vi "SCPI_Log.vi"(11 "SCOP Log In":T1(ring)) -> (3 "SCPI Log Out":string)   [LabVIEW 2009]
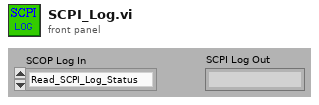
[diagram p1: front panel]
types:
  T1 = enum16{"Read_SCPI_Log_Status", "No_SCPI_Log", "Log_SCPI", "Reset"}
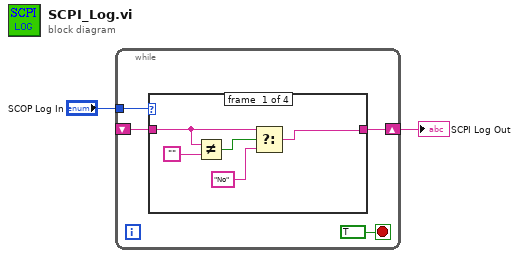
[diagram p0: block diagram]
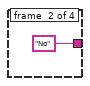
[diagram p2: hidden frame]
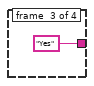
[diagram p3: hidden frame]
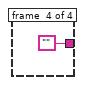
[diagram p4: hidden frame]
diagram:
  n1 = while {
    shift-right: [w5] -> w1
    shift-left: _ -> [w4]
    tunnel: "SCOP Log In" -> [w6]
    stop <- TRUE stop-if-true
    n2 = case shown="\"Read_SCPI_Log_Status\", Default" w6 {
      tunnel: [w8 "No" "Yes" ""] -> w5
      tunnel: w4 -> [w9 _ _ _]
      frame #0 {
        n3 = Not Equal?(x=w9, y="") -> (x != y?=w10:bool)
        n4 = Select(t=w9, s=w10, f="No") -> (s? t:f=w8:string)
      }
      frame #1 {
      }
      frame #2 {
      }
      frame #3 {
      }
    }
  }
  "SCPI Log Out" <- w1
